vi "MagBoard_n128_Serial_Viewer.vi"() -> ()   [LabVIEW 2018]
uses:
  <vilib>/Math Plots/3D Math Plots/3D Surface/3D Surface XCtrl/3D Surface.xctl
  subVIs/calibration/FGVs/FGV States.ctl
  <vilib>/Analysis/baseanly.llb/Mean (DBL).vi
  <vilib>/Utility/file.llb/Write Delimited Spreadsheet (DBL).vi
  <vilib>/Utility/file.llb/Read Delimited Spreadsheet (I64).vi
  <vilib>/Math Plots/3D Math Plots/3D Surface/3D Surface Datatype/Public/Plot Helper (Matrix).vi
  <vilib>/Math Plots/3D Math Plots/3D Surface/3D Surface Datatype/3D Surface Datatype.lvclass
  <vilib>/Analysis/NI_AALBase.lvlib
panel:
  out "Reading":bool
  out "Initialised":bool
  out "Connected":bool
  in  "Tab Control":T1(tab)
  out "3D Surface":refnum<class "3D Plot Datatype.lvclass">[](xcontrol)
  out "Calibrated Output":dbl[][](array[numeric])
  in  "dT":u32=40
  out "Real dT":u32
  out "Initialisation String":string
  out "Data Packet":string
  out "Time":u32=4294745741
  out "Read Count":i32
  out "Lookup Indices":i32[](array[numeric])=[0, 4, 8, 12, 1, 5, 9, 13, 16, 20, 24, 28, 17, 21, 25, 29, 15, 11, 7, 3, 14, 10, 6, 2, 31, 27, 23, 19, 30, 26, 22, 18, 32, 36, 40, 44, 33, 37, 41, 45, 48, 52, 56, 60, 49, 53, 57, 61, 47, 43, 39, 35, 46, 42, 38, 34, 63, 59, 55, 51, 62, 58, 54, 50, 64, 68, 72, 76, 65, 69, 73, 77, 80, 84, 88, 92, 81, 85, 89, 93, 79, 75, 71, 67, 78, 74, 70, 66, 95, 91, 87, 83, 94, 90, 86, 82, 96, 100, 104, 108, 97, 101, 105, 109, 112, 116, 120, 124, 113, 117, 121, 125, 111, 107, 103, 99, 110, 106, 102, 98, 127, 123, 119, 115, 126, 122, 118, 114]
  in  "VISA resource name":refnum<visa-resource-name>="COM16"
  in  "Serial Settings":T2={"baud rate"=115200, "data bits"=8, "parity"=enum."None", "stop bits"=10, "flow control"=0} {"flow control" items=["None"=0, "XON/XOFF"=1, "RTS/CTS"=2, "DTR/DSR"=4]; "stop bits" items=["1.0"=10, "1.5"=15, "2.0"=20]; "data bits" min=5 max=8 step=1; "baud rate" items=["75"=75, "110"=110, "134"=134, "150"=150, "300"=300, "600"=600, "1200"=1200, "1800"=1800, "2400"=2400, "4800"=4800, "7200"=7200, "9600"=9600, "14400"=14400, "19200"=19200, "28800"=28800, "38400"=38400, "56000"=56000, "57600"=57600, "115200"=115200, "128000"=128000, "230400"=230400]}
  in  "Packet Size (Bytes)":u32=1024
  in  "Gains":dbl[](array[numeric])=[0.751, 0.751, 1.21]
  in  "Export File (CSV)":path=path "C:/Users/menprc/Documents/GitHub/MagLib/MagBoard_n64_UI/MagBoard_n64_UI_LabVIEW_Client/example_data/M064_008.csv"
  in  "Save?":bool
  in  "Tare?":bool
  out "Calibrated Output":dbl[][](array[numeric])
  out "B xyz":dbl[][](array[numeric])
  out "Avg X":dbl format="%0.2f"
  out "Avg Y":dbl format="%0.2f"
  in  "stop":bool
  # "ESCAPES:viewer"
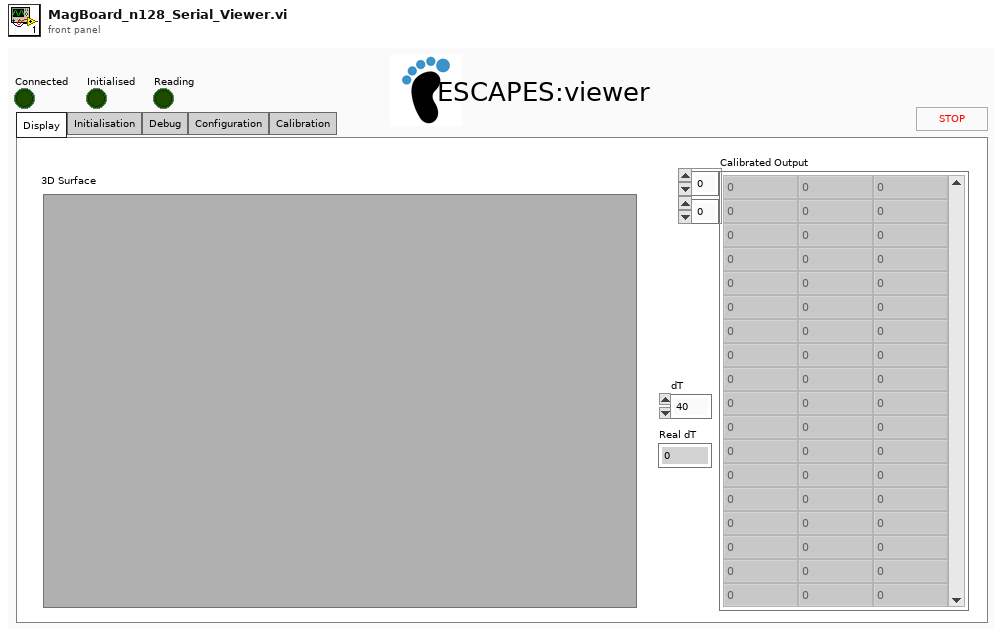
[diagram p1: front panel]
types:
  T1 = enum32{"Display", "Initialisation", "Debug", "Configuration", "Calibration"}
  T2 = cluster{"baud rate":u32, "data bits":u16, "parity":enum16{"None", "Odd", "Even", "Mark", "Space"}, "stop bits":u16, "flow control":u16}
  T3 = typedef "FGV States.ctl" = enum16{"Get", "Set", "Reset"}
  T4 = cluster{cluster{dbl[][], "Array":dbl[][]}, cluster{dbl[][], "Array":dbl[][]}, cluster{dbl[][], "Array":dbl[][]}, cluster{dbl[][], "Array":dbl[][]}}
  T5 = cluster{cluster{dbl[][], "Array":dbl[][]}, cluster{dbl[][], "Array":dbl[][]}, cluster{dbl[][], "Array":dbl[][]}, cluster{dbl[][], "Array":dbl[][]}}[]
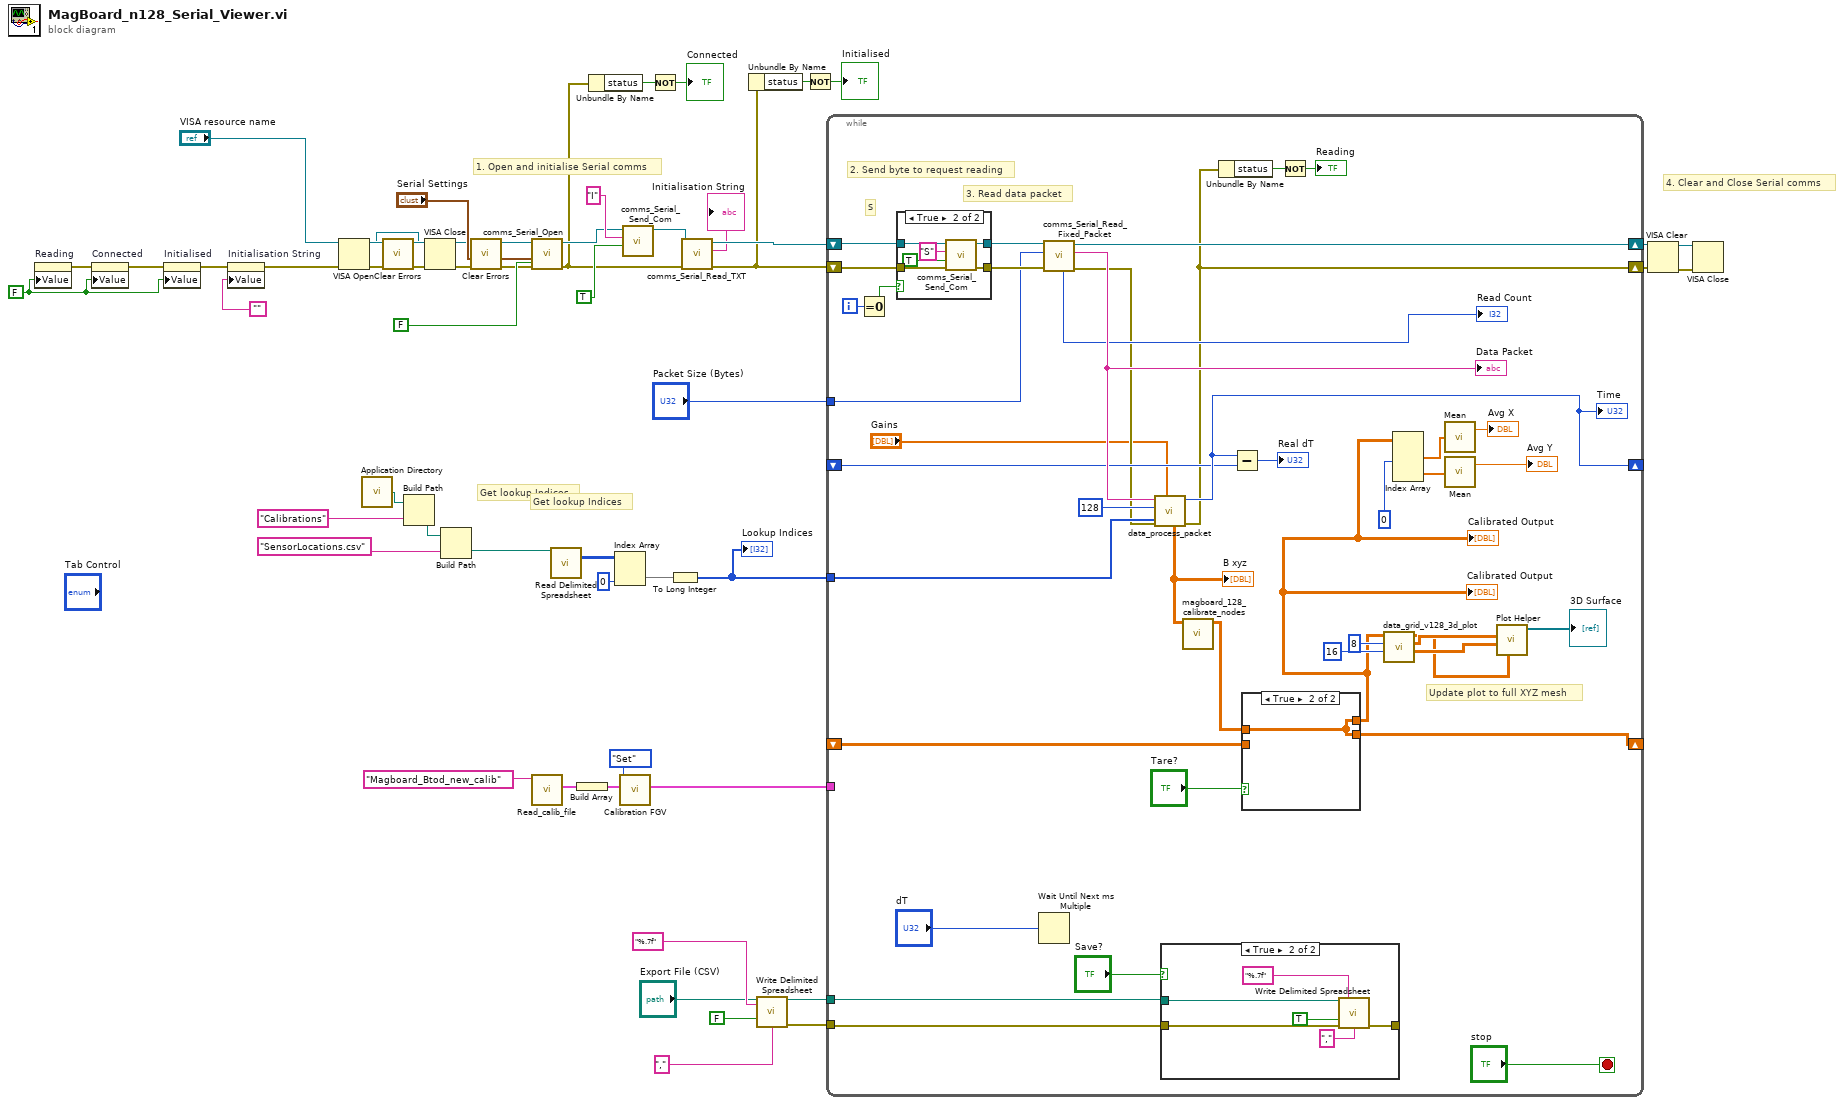
[diagram p0: block diagram]
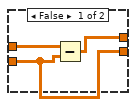
[diagram p2: hidden frame]
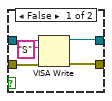
[diagram p4: hidden frame]
diagram:
  w27 = FALSE ("Send Init Comm?")
  # "Get lookup Indices"
  # "Get lookup Indices"
  # "4. Clear and Close Serial comms"
  # "1. Open and initialise Serial comms"
  n1 = property on="Reading" class="Bool (strict)"("Value"=w27) -> (error out=w29:errorcluster)  [unwired: 2 in, 1 out]
  n2 = property on="Connected" class="Bool (strict)"(error in=w29, "Value"=w27) -> (error out=w30:errorcluster)  [unwired: 1 in, 1 out]
  n3 = property on="Initialised" class="Bool (strict)"(error in=w30, "Value"=w27) -> (error out=w28:errorcluster)  [unwired: 1 in, 1 out]
  n4 = property on="Initialisation String" class="Str"(error in=w28, "Value"="") -> (error out=w20:errorcluster)  [unwired: 1 in, 1 out]
  n5 = VISA Open(error in (no error)=w20, VISA resource name="VISA resource name") -> (VISA resource name=w18:refnum<visa-resource-name>, error out=w17:errorcluster)  [unwired: 3 in]
  n6 = call <vilib>:"Application Directory.vi"() -> ("Application Directory"=w2:path)
  n7 = call <vilib>:"Clear Errors.vi"("error in (no error)"=w17) -> ("error out"=w16:errorcluster)  [unwired: 5 in, 1 out]
  n8 = Build Path(base path=w2, name or relative path="Calibrations" ("string")) -> (appended path=w4:path)
  n9 = VISA Close(VISA resource name=w18, error in (no error)=w16) -> (error out=w15:errorcluster)
  n10 = Build Path(base path=w4, name or relative path="SensorLocations.csv" ("string")) -> (appended path=w1:path)
  n11 = call <vilib>:"Clear Errors.vi"("error in (no error)"=w15) -> ("error out"=w14:errorcluster)  [unwired: 5 in, 1 out]
  n12 = call "comms_Serial_Open.vi"("Send Init Comm?"=FALSE, "error in (no error)"=w14, "Serial Settings in"="Serial Settings", "VISA Refnum in"="VISA resource name") -> ("error out"=w36:errorcluster, "VISA Refnum out"=w43:refnum<visa-resource-name>)  [unwired: 5 in, 1 out]
  n13 = call "Read_calib_file.vi"("string"="Magboard_Btod_new_calib" ("Command")) -> ("output cluster"=w9:T4)  [unwired: 6 in, 4 out]
  n14 = call-poly <vilib>:"Read Delimited Spreadsheet.vi"("file path (dialog if empty)"=w1) -> ("all rows"=w13:i64[][])  [unwired: 9 in, 5 out]
  n15 = Build Array(w9) -> (w8:T5)
  n16 = Unbundle By Name(w36) -> ("status"=w35:bool)
  n17 = Index Array(array=w13, index (col)=0 ("disabled index (col)")) -> (element=w11:i64[])  [unwired: 1 in]
  n18 = call "Calibration FGV.vi"("Calib in"=w8, "FGV States"=FGV_States."Set") -> ("Calib in 2"=w6:T5)  [unwired: 9 in]
  n19 = call "comms_Serial_Send_Com.vi"("Buffer Clear?"=TRUE, "Command"="I", "VISA resource in"=w43) -> ("VISA resource Out"=w41:refnum<visa-resource-name>)  [unwired: 6 in, 2 out]
  n20 = Not(x=w35) -> (.not. x?=→"Connected":bool)
  n21 = To Long Integer(number=w11) -> (32bit integer=w37:i32[])
  "Lookup Indices" <- w37
  n22 = call "comms_Serial_Read_TXT.vi"("error in"=w36, "VISA resource in"=w41) -> ("error out"=w33:errorcluster, "Data Out"=→"Initialisation String":string, "VISA resource Out"=w40:refnum<visa-resource-name>)  [unwired: 6 in, 1 out]
  n23 = Unbundle By Name(w33) -> ("status"=w34:bool)
  n24 = call-poly <vilib>:"Write Delimited Spreadsheet.vi"("file path (dialog if empty)"="Export File (CSV)", "format (%.3f)"="%.7f", "append to file? (new file:F)"=FALSE, "delimiter (\\t)"="," ("delimiter (\\t)")) -> ("new file path (Not A Path if cancelled)"=w22:path, "error out"=w21:errorcluster)  [unwired: 10 in]
  n25 = Not(x=w34) -> (.not. x?=→"Initialised":bool)
  n26 = while {
    shift-right: [w83] -> w46
    shift-left: w40 -> [w89]
    tunnel: w37 -> [w90]
    shift-right: [w73] -> w45
    shift-left: w33 -> [w88]
    tunnel: "Packet Size (Bytes)" -> [w81]
    shift-right: [w78] -> _
    shift-left: _ -> [w77]
    tunnel: w22 -> [w71]
    tunnel: w21 -> [w70]
    tunnel: w6 -> [_]
    shift-right: [w64] -> _
    shift-left: _ -> [w66]
    i -> [w87]
    stop <- "stop" stop-if-true
    # "Update plot to full XYZ mesh"
    # "3. Read data packet"
    # "2. Send byte to request reading"
    # "S"
    n27 = Equal To 0?(x=w87) -> (x = 0?=w79:bool)
    n28 = case shown="True" w79 {
      tunnel: w89 -> [w109 w115]
      tunnel: w88 -> [w106 w113]
      tunnel: [w108 w112] -> w85
      tunnel: [w105 w111] -> w84
      frame False {
        n29 = VISA Write(VISA resource name=w109, write buffer="S", error in (no error)=w106) -> (VISA resource name out=w108:refnum<visa-resource-name>, error out=w105:errorcluster)  [unwired: 1 out]
      }
      frame True {
        n30 = call "comms_Serial_Send_Com.vi"("error in"=w113, "Buffer Clear?"=TRUE, "Command"="S", "VISA resource in"=w115) -> ("error out"=w111:errorcluster, "VISA resource Out"=w112:refnum<visa-resource-name>)  [unwired: 5 in, 1 out]
      }
    }
    n31 = Wait Until Next ms Multiple(millisecond multiple="dT") -> ()  [unwired: 1 out]
    n32 = call "comms_Serial_Read_Fixed_Packet.vi"("error in"=w84, "Packet Size (Bytes)"=w81, "VISA resource in"=w85) -> ("error out"=w75:errorcluster, "Data Out"=w82:string, "VISA resource Out"=w83:refnum<visa-resource-name>, "Bytes Read"=→"Read Count":u32)  [unwired: 4 in, 1 out]
    "Data Packet" <- w82
    n33 = call "data_process_packet.vi"("Sensor Lookup Indices"=w90, "Gains"="Gains", "error in (no error)"=w75, "No. Sensors"=128 ("No. Nodes"), "Binary Input Data"=w82) -> ("error out"=w73:errorcluster, "Time"=w78:u32, "Sensors (uT)"=w68:dbl[][])  [unwired: 2 in, 2 out]
    "Time" <- w78
    "B xyz" <- w68
    n34 = case shown="True" "Save?" {
      tunnel: w71 -> [_ w101]
      tunnel: w70 -> [w98 w100]
      tunnel: [w98 w99] -> _
      frame False {
      }
      frame True {
        n35 = call-poly <vilib>:"Write Delimited Spreadsheet.vi"("file path (dialog if empty)"=w101, "format (%.3f)"="%.7f", "append to file? (new file:F)"=TRUE, "error in (no error)"=w100, "delimiter (\\t)"="," ("delimiter (\\t)")) -> ("error out"=w99:errorcluster)  [unwired: 9 in, 1 out]
      }
    }
    n36 = call "magboard_128_calibrate_nodes.vi"("Sensor Input (mT)"=w68) -> ("Sensor Output - Position (mm)"=w63:dbl[][])  [unwired: 10 in]
    n37 = Unbundle By Name(w73) -> ("status"=w74:bool)
    n38 = Subtract(x=w78, y=w77) -> (x-y=→"Real dT":u32)
    n39 = case shown="True" "Tare?" {
      tunnel: w63 -> [w96 w97]
      tunnel: w66 -> [w95 _]
      tunnel: [w95 w97] -> w64
      tunnel: [w94 w97] -> w57
      frame False {
        n40 = Subtract(x=w96, y=w95) -> (x-y=w94:dbl[][])
      }
      frame True {
      }
    }
    "Calibrated Output" <- w57
    "Calibrated Output" <- w57
    n41 = Not(x=w74) -> (.not. x?=→"Reading":bool)
    n42 = call "data_grid_v128_3d_plot.vi"("No. Rows"=16 ("Row Length"), "No. Columns"=8, "Sensor Data"=w57) -> ("Y (GRID)"=w59:dbl[][], "X (GRID)"=w60:dbl[][], "Z (GRID)"=w58:dbl[][])  [unwired: 6 in]
    n43 = Index Array(array=w57, index (col) #1=0 ("disabled index (col)")) -> (element #1=w54:dbl[], element #2=w55:dbl[])  [unwired: 3 in]
    n44 = call-poly <vilib>:"Mean.vi"("X"=w54) -> ("mean"=→"Avg X":dbl)  [unwired: 1 out]
    n45 = call-poly <vilib>:"Mean.vi"("X"=w55) -> ("mean"=→"Avg Y":dbl)  [unwired: 1 out]
    n46 = call-poly <vilib>:"Plot Helper.vi"("z matrix"=w58, "y matrix"=w59, "x matrix"=w60) -> ("3D Plot lvclass Array out"=→"3D Surface":refnum<class "3D Plot Datatype.lvclass">[])  [unwired: 3 in, 5 out]
  }
  n47 = VISA Clear(VISA resource name=w46, error in (no error)=w45) -> (VISA resource name out=w48:refnum<visa-resource-name>, error out=w47:errorcluster)
  n48 = VISA Close(VISA resource name=w48, error in (no error)=w47) -> ()  [unwired: 1 out]
